vi "Drive Motor Controler.vi"   [LabVIEW 2009]
uses:
  Motor Output Global.vi
  Drive Control Global DO NOT MODIFY!.vi
  Motor Encoder Global.vi
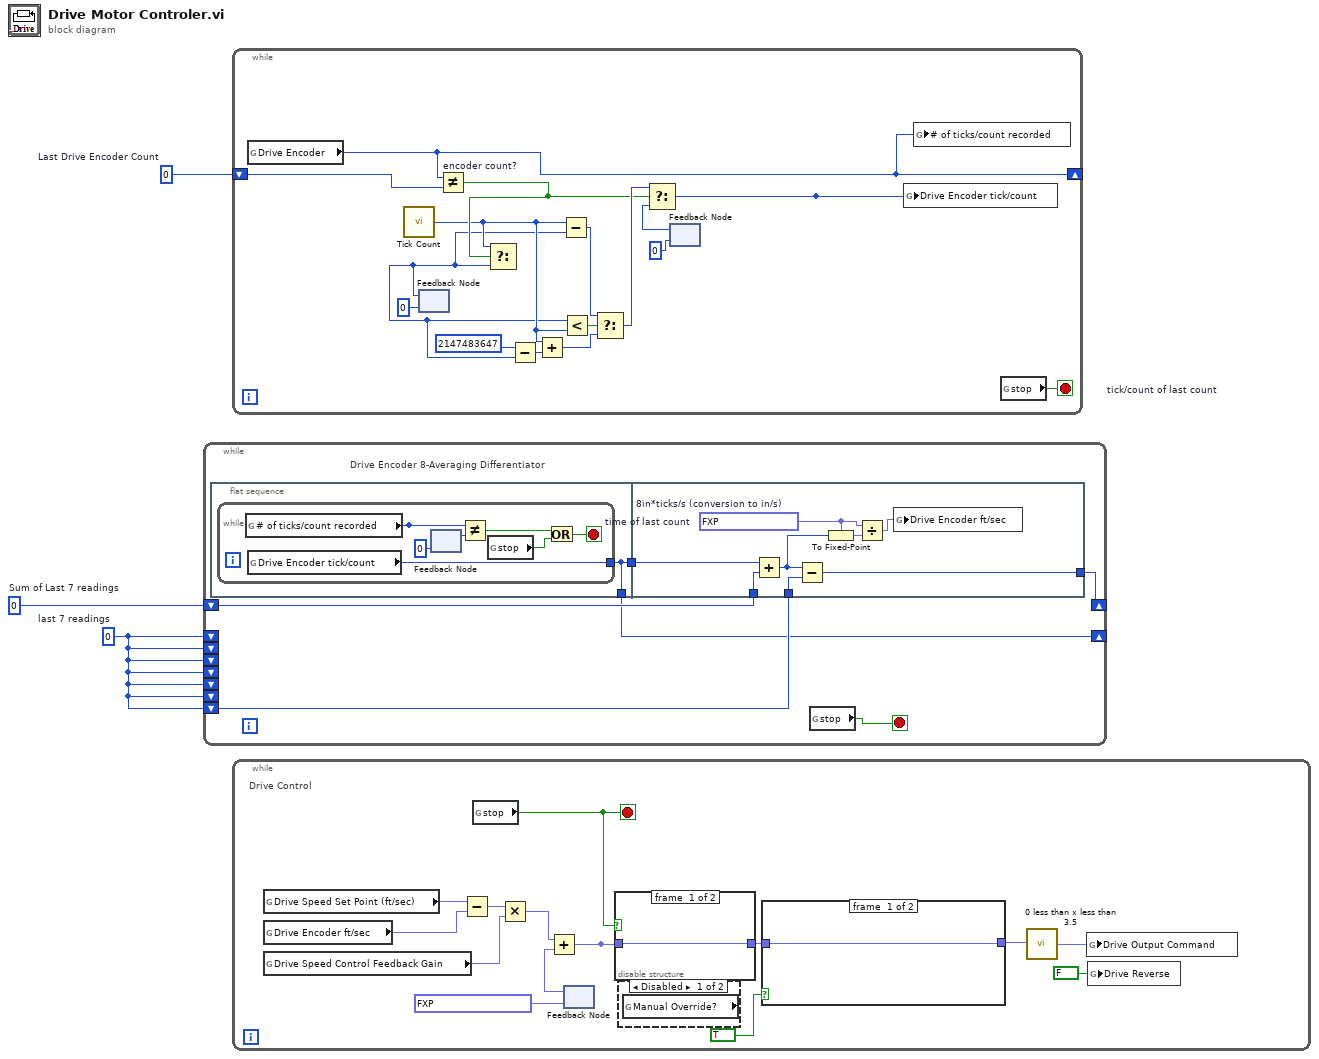
[diagram p0: block diagram]
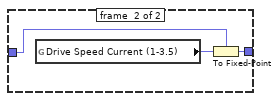
[diagram p3: hidden frame]
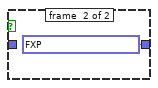
[diagram p4: hidden frame]
diagram:
  w1 = 0  # Last Drive Encoder Count
  w2 = u32 0  # last 7 readings
  w3 = u32 0  # Sum of Last 7 readings
  n1 = while {
    shift-right: [w9] -> _
    shift-left: w3 -> [w6]
    shift-right: [w4] -> _
    shift-left: w2 -> [_]
    shift-left: w2 -> [_]
    shift-left: w2 -> [_]
    shift-left: w2 -> [_]
    shift-left: w2 -> [_]
    shift-left: w2 -> [_]
    shift-left: w2 -> [w8]
    stop <- w5 stop-if-true
    # "Drive Encoder 8-Averaging Differentiator"
    n2 = flat-sequence {
      tunnel: [w10] -> w7
      tunnel: [w10] -> w4
      tunnel: [w23] -> w9
      tunnel: w8 -> [w22]
      tunnel: w7 -> [w21]
      tunnel: w6 -> [w20]
      frame #0 {
        n3 = while {
          tunnel: [w15] -> w10
          stop <- w11 stop-if-true
          n4 = global read "Drive Control Global DO NOT MODIFY!.vi" "# of ticks/count recorded"() -> (w14:i32)
          n5 = global read "Drive Control Global DO NOT MODIFY!.vi" "Drive Encoder tick/count"() -> (w15:u32)
          n6 = feedback #1(0 ("Drive Encoder tick/count")) -> (w17:i32)
          n7 = Not Equal?(x=w14, y=w17) -> (x != y?=w12:bool)
          n8 = global read "Motor Encoder Global.vi" "stop"() -> (w13:bool)
          n9 = Or(x=w12, y=w13) -> (x .or. y?=w11:bool)
        }
      }
      frame #1 {
        w18 = fxp<+,31,21> 1387360.33984375  # 8in*ticks/s (conversion to in/s)
        n10 = Add(x=w21, y=w20) -> (x+y=w24:u32)
        n11 = Subtract(x=w24, y=w22) -> (x-y=w23:u32)
        n12 = To Fixed-Point(fixed-point type=w18, number=w24) -> (fixed-point=w25:fxp<+,31,21>)
        n13 = Divide(x=w18, y=w25) -> (x/y=w19:fxp<+/-,18,8>)
        n14 = global write "Drive Control Global DO NOT MODIFY!.vi" "Drive Encoder ft/sec"(w19) -> ()
      }
    }
    n15 = global read "Motor Encoder Global.vi" "stop"() -> (w5:bool)
  }
  n16 = while {
    shift-right: [w39] -> _
    shift-left: w1 -> [w40]
    stop <- w41 stop-if-true
    n17 = global read "Motor Encoder Global.vi" "Drive Encoder"() -> (w39:i32)
    n18 = call "Tick Count"() -> ("Tick Count(Ticks)"=w29:u32)
    n19 = feedback #2 "time of last count"(u32 0 ("Tick Count(Ticks)")) -> (w26:u32)
    n20 = Not Equal? "encoder count?"(x=w39, y=w40) -> (x != y?=w30:bool)
    n21 = Select(t=w29, s=w30, f=w26) -> (s? t:f=w27:u32)
    n22 = Subtract(x=u32 2147483647, y=w26) -> (x-y=w37:u32)
    n23 = Add(x=w29, y=w37) -> (x+y=w35:u32)
    n24 = Subtract(x=w29, y=w26) -> (x-y=w36:u32)
    n25 = Less?(x=w26, y=w29) -> (x < y?=w31:bool)
    n26 = Select(t=w36, s=w31, f=w35) -> (s? t:f=w34:u32)
    n27 = feedback #3 "tick/count of last count"(u32 0) -> (w33:u32)
    n28 = Select(t=w34, s=w30, f=w33) -> (s? t:f=w42:u32)
    n29 = global write "Drive Control Global DO NOT MODIFY!.vi" "Drive Encoder tick/count"(w42) -> ()
    n30 = global write "Drive Control Global DO NOT MODIFY!.vi" "# of ticks/count recorded"(w39) -> ()
    n31 = global read "Motor Encoder Global.vi" "stop"() -> (w41:bool)
  }
  n32 = while {
    stop <- w52 stop-if-true
    # "Drive Control"
    n33 = global read "Motor Encoder Global.vi" "Drive Speed Set Point (ft/sec)"() -> (w54:fxp<+/-,18,8>)
    n34 = global read "Drive Control Global DO NOT MODIFY!.vi" "Drive Encoder ft/sec"() -> (w55:fxp<+/-,18,8>)
    n35 = global read "Motor Encoder Global.vi" "Drive Speed Control Feedback Gain"() -> (w53:fxp<+/-,13,4>)
    n36 = Subtract(x=w54, y=w55) -> (x-y=w56:fxp<+/-,20,5>)
    n37 = global read "Motor Encoder Global.vi" "stop"() -> (w52:bool)
    n38 = Multiply(x=w56, y=w53) -> (x*y=w47:fxp<+/-,20,5>)
    n39 = feedback #4(fxp<+/-,20,5> 0.0 ("coerced x")) -> (w46:fxp<+/-,20,5>)
    n40 = Add(x=w47, y=w46) -> (x+y=w44:fxp<+/-,20,5>)
    n41 = case shown="False" w52 {
      tunnel: w44 -> [w61 _]
      tunnel: [w61 fxp<+/-,20,5> 0.0] -> w51
      frame #0 {
      }
      frame #1 {
      }
    }
    n42 = disable-structure shown="Disabled" {
      frame #0 {
        n43 = global read "Motor Output Global.vi" "Manual Override?"() -> ()  [unwired: 1 out]
      }
      frame #1 {
      }
    }
    n44 = case shown="True" TRUE {
      tunnel: [w57 w59] -> w50
      tunnel: w51 -> [w57 w58]
      frame #0 {
      }
      frame #1 {
        n45 = global read "Motor Encoder Global.vi" "Drive Speed Current (1-3.5)"() -> (w60:fxp<+/-,18,8>)
        n46 = To Fixed-Point(fixed-point type=w58, number=w60) -> (fixed-point=w59:fxp<+/-,20,5>)
      }
    }
    n47 = call "0 less than x less than 3.5.vi"("x"=w50) -> ("coerced x"=w49:fxp<+/-,20,5>)
    n48 = global write "Motor Output Global.vi" "Drive Output Command"(w49) -> ()
    n49 = global write "Motor Output Global.vi" "Drive Reverse"(FALSE ("Drive Reverse")) -> ()
  }
